vi "front Sw--P cube1.vi"(1 "F-Sw--F-Cube":T1, 3 "Command Info In":T2, 4 "Switch":string) -> (10 "Command Info Out":T2)   [LabVIEW 2017]
uses:
  <vilib>/Rock Robotics/WPI/Framework/Command Status Info.ctl
  <vilib>/Rock Robotics/WPI/Framework/Completion Status.ctl
  <vilib>/Rock Robotics/WPI/Framework/Completion Notifier.ctl
  Block Clusters/front Sw--P cube1.ctl
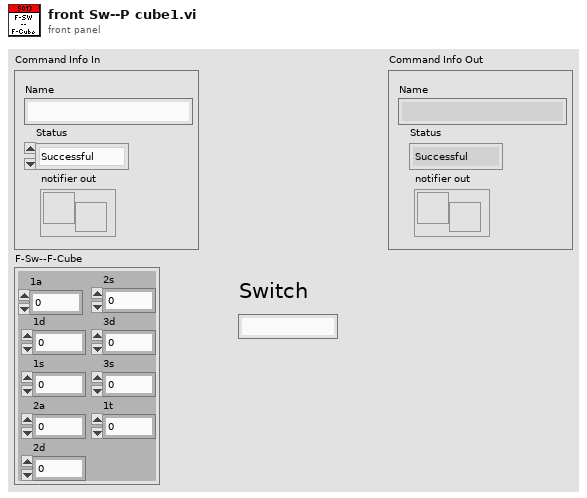
[diagram p1: front panel]
types:
  T1 = typedef "front Sw--P cube1.ctl" = cluster{"1a":dbl, "1d":dbl, "1s":dbl, "2a":dbl, "2d":dbl, "2s":dbl, "3d":dbl, "3s":dbl, "1t":dbl}
  T2 = typedef "Command Status Info.ctl" = cluster{"Name":string, "Status":T3, "notifier out":T4}
  T3 = typedef "Completion Status.ctl" = enum16{"Successful", "Aborted", "Incomplete"}
  T4 = typedef "Completion Notifier.ctl" = refnum<notifier>
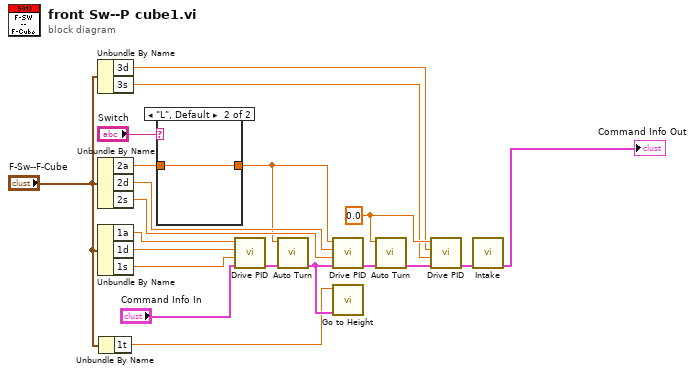
[diagram p0: block diagram]
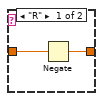
[diagram p2: hidden frame]
diagram:
  w11 = 0.0 ("Target Angle")
  n1 = Unbundle By Name("F-Sw--F-Cube") -> ("3d"=w9:dbl, "3s"=w8:dbl)
  n2 = Unbundle By Name("F-Sw--F-Cube") -> ("2a"=w4:dbl, "2d"=w13:dbl, "2s"=w5:dbl)
  n3 = Unbundle By Name("F-Sw--F-Cube") -> ("1a"=w2:dbl, "1d"=w15:dbl, "1s"=w14:dbl)
  n4 = Unbundle By Name("F-Sw--F-Cube") -> ("1t"=w6:dbl)
  n5 = case shown="\"L\", Default" "Switch" {
    tunnel: [w21 w23] -> w1
    tunnel: w4 -> [w22 w23]
    frame "R" {
      n6 = Negate(x=w22) -> (-x=w21:dbl)
    }
    frame "L", Default {
    }
  }
  n7 = call "Drive PID.vi"("Command Info In"="Command Info In", "Speed"=w14, "Distance"=w15, "Target Angle"=w2) -> ("Command Info Out"=w20:T2)  [unwired: 7 in]
  n8 = call "Auto Turn.vi"("Command Info In"=w20, "Target Angle"=w1) -> ("Command Info Out"=w17:T2)  [unwired: 9 in]
  n9 = call "Drive PID.vi"("Command Info In"=w17, "Speed"=w5, "Distance"=w13, "Target Angle"=w1) -> ("Command Info Out"=w16:T2)  [unwired: 7 in]
  n10 = call "Go to Height.vi"("Command Info In"=w17, "Target Height (in)"=w6) -> ()  [unwired: 9 in, 1 out]
  n11 = call "Auto Turn.vi"("Command Info In"=w16, "Target Angle"=w11) -> ("Command Info Out"=w12:T2)  [unwired: 9 in]
  n12 = call "Drive PID.vi"("Command Info In"=w12, "Speed"=w8, "Distance"=w9, "Target Angle"=w11) -> ("Command Info Out"=w10:T2)  [unwired: 7 in]
  n13 = call "Intake.vi"("Command Info In"=w10) -> ("Command Info Out"=→"Command Info Out":T2)  [unwired: 10 in]
